vi "text_editor.vi"() -> ()   [LabVIEW 2019]
panel:
  in  "Write":bool
  in  "Read":bool
  in  "Stop":bool
  in  "file path":path
  out "error out":errorcluster
  in  "Text":string
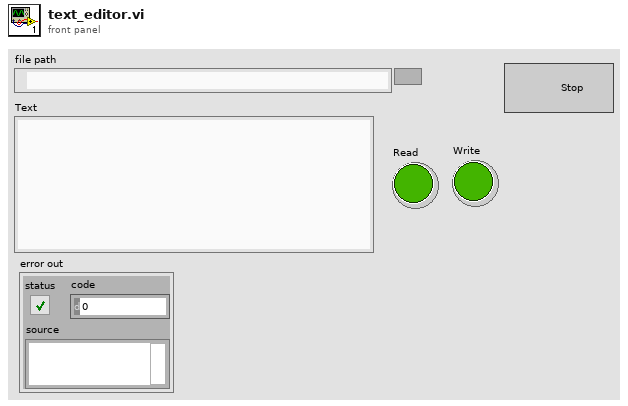
[diagram p1: front panel]
types:
  T1 = enum16{"open", "replace", "create", "open or create", "replace or create", "replace or create with confirmation"}
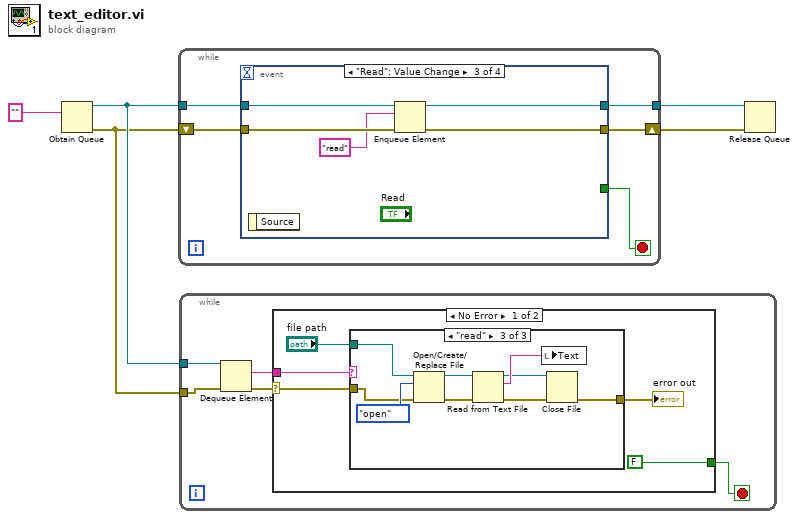
[diagram p0: block diagram]
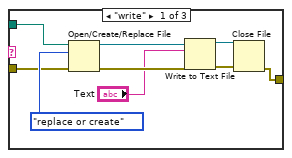
[diagram p2: hidden frame]
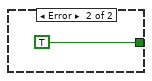
[diagram p4: hidden frame]
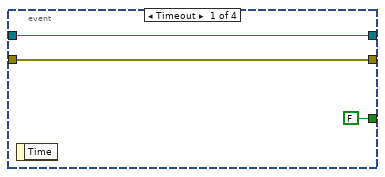
[diagram p5: hidden frame]
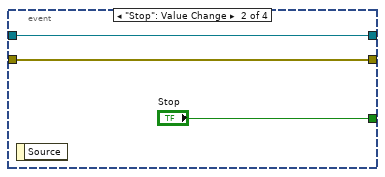
[diagram p6: hidden frame]
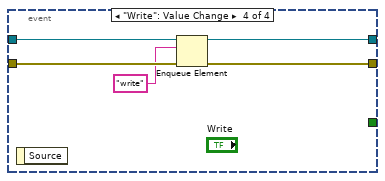
[diagram p7: hidden frame]
diagram:
  n1 = Obtain Queue(element data type="") -> (queue out=w2:refnum<queue>, error out=w1:errorcluster)  [unwired: 4 in, 1 out]
  n2 = while {
    tunnel: w2 -> [w8]
    shift-right: [w7] -> w4
    shift-left: w1 -> [w9]
    tunnel: [w6] -> w3
    stop <- w10 stop-if-true
    n3 = event shown="[2] \"Read\": Value Change" {
      selector: _ -> [_ _ _ _]
      dyn-events: _ -> [_ _ _ _]
      timeout: _ -> [_ _ _ _]
      tunnel: [FALSE ("Stop") "Stop" _ _] -> w10
      tunnel: w9 -> [w12 w15 w21 w26]
      tunnel: w8 -> [w11 w14 w20 w24]
      tunnel: [w12 w15 w19 w25] -> w7
      tunnel: [w11 w14 w18 w23] -> w6
      event Timeout {
        n4 = event-data() -> ()  [unwired: 1 in, 1 out]
      }
      event "Stop": Value Change {
        n5 = event-data() -> ()  [unwired: 1 in, 1 out]
      }
      event "Read": Value Change {
        n6 = event-data() -> ()  [unwired: 1 in, 1 out]
        n7 = Enqueue Element(queue=w20, element="read", error in (no error)=w21) -> (queue out=w18:refnum<queue>, error out=w19:errorcluster)  [unwired: 1 in, 1 out]
      }
      event "Write": Value Change {
        n8 = event-data() -> ()  [unwired: 1 in, 1 out]
        n9 = Enqueue Element(queue=w24, element="write", error in (no error)=w26) -> (queue out=w23:refnum<queue>, error out=w25:errorcluster)  [unwired: 1 in, 1 out]
      }
    }
  }
  n10 = while {
    tunnel: w2 -> [w31]
    tunnel: w1 -> [w30]
    stop <- w28 stop-if-true
    n11 = Dequeue Element(queue=w31, error in (no error)=w30) -> (element=w27:string, error out=w29:errorcluster)  [unwired: 1 in, 2 out]
    n12 = case shown="No Error" w29 {
      selector: w29 -> [w34 _]
      tunnel: [FALSE TRUE] -> w28
      tunnel: w27 -> [w35 _]
      frame No Error {
        n13 = case shown="\"read\"" w35 {
          tunnel: "file path" -> [w44 _ w55]
          tunnel: w34 -> [w43 w46 w52]
          tunnel: [w37 w46 w47] -> w33
          frame "write" {
            n14 = Open/Create/Replace File(file path (use dialog)=w44, error in=w43, operation (0:open)=T1."replace or create") -> (refnum out=w41:refnum<file>, error out=w42:errorcluster)  [unwired: 3 in, 1 out]
            n15 = Write to Text File(file (use dialog)=w41, text="Text", error in=w42) -> (refnum out=w38:refnum<file>, error out=w39:errorcluster)  [unwired: 1 in, 1 out]
            n16 = Close File(refnum=w38, error in=w39) -> (error out=w37:errorcluster)  [unwired: 1 out]
          }
          frame Default {
          }
          frame "read" {
            n17 = Open/Create/Replace File(file path (use dialog)=w55, error in=w52, operation (0:open)=T1."open") -> (refnum out=w54:refnum<file>, error out=w51:errorcluster)  [unwired: 3 in, 1 out]
            n18 = Read from Text File(file (use dialog)=w54, error in=w51) -> (refnum out=w48:refnum<file>, text=w50:string, error out=w49:errorcluster)  [unwired: 2 in, 1 out]
            n19 = local write "Text"(w50) -> ()
            n20 = Close File(refnum=w48, error in=w49) -> (error out=w47:errorcluster)  [unwired: 1 out]
          }
        }
        "error out" <- w33
      }
      frame Error {
      }
    }
  }
  n21 = Release Queue(queue=w3, error in (no error)=w4) -> ()  [unwired: 1 in, 3 out]
